vi "Get diagnostic value.vi"(8 "error in (no error)":errorcluster, 10 "X command (X8)":u16(ring)=8 items=["X0 - Zero Cal Store", "X1 - Gain Cal Store", "X2 - STD Cal Gain Factor", "X3 - Zero Offset", "X4 - Gain Offset", "X5 - Linearity", "X6 - Reference Divider Setting", "X7 - Spot Freq. Corrections", "X8 - User Message Recall", "X9 - Recall Cal Store Selection"], 11 "VISA resource name":refnum<visa-resource-name>) -> (0 "error out":errorcluster, 1 "Respond string":string, 2 "Respond number":dbl, 3 "VISA resource name out":refnum<visa-resource-name>)   [LabVIEW 2012, in "Datron D4xxx.lvlib"]
doc: "This VI sends X command and returns respond string and its covnersion to number if possible."
uses:
  Datron D4xxx.lvlib
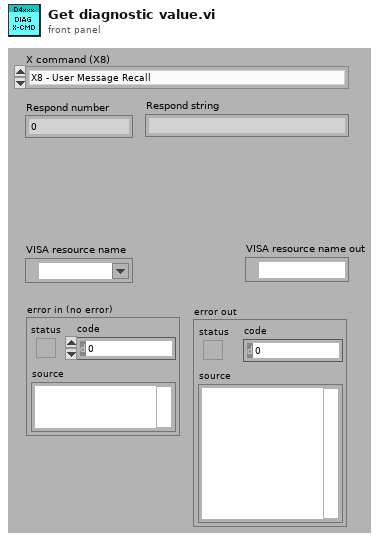
[diagram p1: front panel]
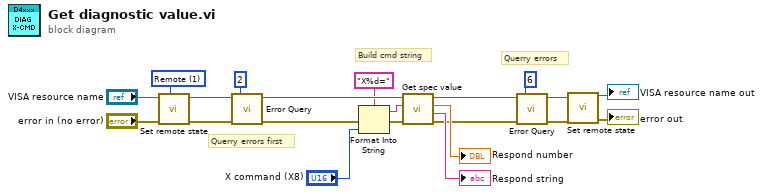
[diagram p0: block diagram]
diagram:
  w19 = u16 1 items=["Local", "Remote", "Default"] ("Remote state")
  # "Querry errors"
  # "Querry errors first"
  # "Build cmd string"
  n1 = call "Set remote state.vi"("error in"="error in (no error)", "Remote state"=w19, "VISA resource name"="VISA resource name") -> ("error out"=w16:errorcluster, "VISA resource name out"=w15:refnum<visa-resource-name>)  [unwired: 7 in]
  n2 = call "Error Query.vi"("error in (no error)"=w16, "Check cycles (11)"=2, "VISA resource name"=w15) -> ("error out"=w4:errorcluster, "VISA resource name out"=w13:refnum<visa-resource-name>)  [unwired: 5 in, 2 out]
  n3 = Format Into String(format string="X%d=", error in=w4, "X command (X8)") -> (resulting string=w3:string, error out=w5:errorcluster)  [unwired: 1 in]
  n4 = call "Get spec value.vi"("error in (no error)"=w5, "Command string"=w3, "VISA resource name"=w13) -> ("error out"=w6:errorcluster, "Value string"=→"Respond string":string, "Value"=→"Respond number":dbl, "VISA resource name out"=w7:refnum<visa-resource-name>)  [unwired: 5 in]
  n5 = call "Error Query.vi"("error in (no error)"=w6, "Check cycles (11)"=6, "VISA resource name"=w7) -> ("error out"=w9:errorcluster, "VISA resource name out"=w10:refnum<visa-resource-name>)  [unwired: 5 in, 2 out]
  n6 = call "Set remote state.vi"("error in"=w9, "VISA resource name"=w10) -> ("error out"=→"error out":errorcluster, "VISA resource name out"=→"VISA resource name out":refnum<visa-resource-name>)  [unwired: 8 in]
